vi "Perform Action.vi"(8 "error in":errorcluster, 10 "Input":variant, 11 "Virt Instrument Base in":refnum<class "Virt Instr Target Gain.lvclass">) -> (0 "error out":errorcluster, 2 "Output":variant, 3 "Virt Instrument Base out":refnum<class "Virt Instr Target Gain.lvclass">)   [LabVIEW 2023, in "HAL GOOP4.lvlib" / "Virt Instr Target Gain.lvclass"]
uses:
  Virt Instr Target Gain.lvclass
  Virt Instr Target Gain.lvclass/Virt Instr Target Gain.ctl
  Virt Instr Base/Virt Instr Base.lvclass
  af659c39-85a5-447e-8f09-7029c30334c7.vi
  <userlib>/_OpenG.lib/lvdata/lvdata.llb/openg_variant.lvlib
  Virt Instr Target/Virt Instr Target.lvclass
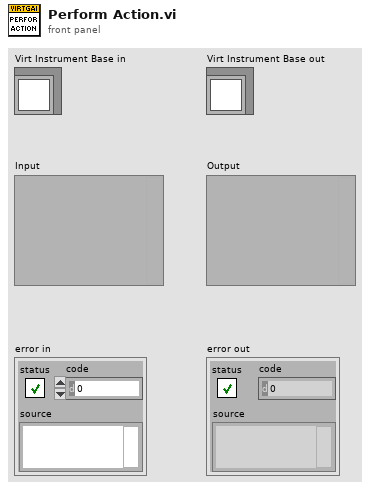
[diagram p1: front panel]
types:
  T1 = typedef "openg_variant.lvlib/Type Descriptor Enumeration__ogtk.ctl" = enum8{"<Null>", "I8", "I16", "I32", "I64", "U8", "U16", "U32", "U64", "SGL", "DBL", "EXT", "CSG", "CDB", "CXT", "0x0F", "0x10", "0x11", "0x12", "0x13", "0x14", "Enum U8", "Enum U16", "Enum U32", "Enum U64", "SGL PQ", "DBL PQ", "EXT PQ", "CSG PQ", "CDB PQ", "CXT PQ", "0x1F", "0x20", "Boolean", "0x22", "0x23", "0x24", "0x25", "0x26", "0x27", "0x28", "0x29", "0x2A", "0x2B", "0x2C", "0x2D", "0x2E", "0x2F", "String", "0x31", "Path", "Pict", "0x34", "0x35", "0x36", "DAQ", "0x38", "0x39", "0x3A", "0x3B", "0x3C", "0x3D", "0x3E", "0x3F", "Array", "0x41", "0x42", "0x43", "0x44", "0x45", "0x46", "0x47", "0x48", "0x49", "0x4A", "0x4B", "0x4C", "0x4D", "0x4E", "0x4F", "Cluster", "0x51", "0x52", "Variant", "Waveform", "0x55", "0x56", "0x57", "0x58", "0x59", "0x5A", "0x5B", "0x5C", "0x5D", "0x5E", "Fixed Point", "0x60", "0x61", "0x62", "0x63", "0x64", "0x65", "0x66", "0x67", "0x68", "0x69", "0x6A", "0x6B", "0x6C", "0x6D", "0x6E", "0x6F", "Refnum", "0x71", "0x72", "Set Collection", "Map Collection"}
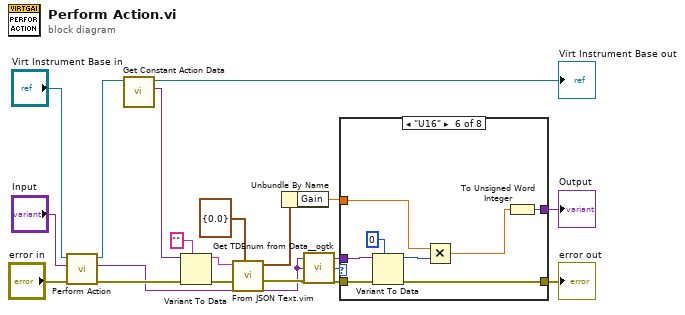
[diagram p0: block diagram]
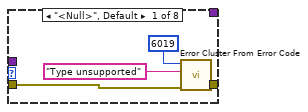
[diagram p2: hidden frame]
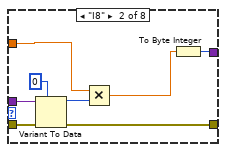
[diagram p3: hidden frame]
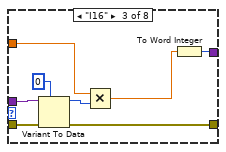
[diagram p4: hidden frame]
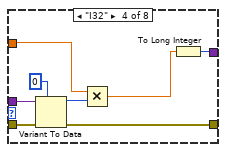
[diagram p5: hidden frame]
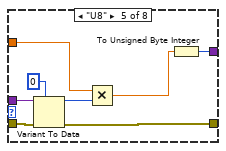
[diagram p6: hidden frame]
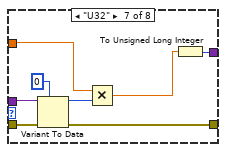
[diagram p7: hidden frame]
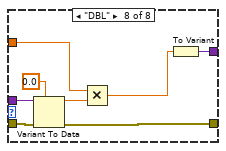
[diagram p8: hidden frame]
diagram:
  n1 = call-parent "Perform Action.vi"("error in"="error in", "Input"="Input", "Virt Instrument Base in"="Virt Instrument Base in") -> ("error out"=w5:errorcluster, "Output"=w3:variant, "Virt Instrument Base out"=w18:refnum<class "Virt Instr Target Gain.lvclass">)  [unwired: 6 in]
  n2 = call "Get Constant Action Data.vi"("Virt Instr Base in"=w18) -> ("Constant Action Data"=w12:variant, "Virt Instr Base out"=→"Virt Instrument Base out":refnum<class "Virt Instr Target Gain.lvclass">)  [unwired: 9 in]
  n3 = Variant To Data(error in=w5, type="", Variant=w12) -> (data=w11:string, error out=w10:errorcluster)
  n4 = call "From JSON Text.vim"("Data Type and Default Value"=cluster{"Gain":dbl} {"Gain"=0.0}, "error in (no error)"=w10, "JSON"=w11) -> ("error out"=w7:errorcluster, "Data out"=w8:cluster{"Gain":dbl})  [unwired: 7 in]
  n5 = Unbundle By Name(w8) -> ("Gain"=w6:dbl)
  n6 = call <userlib>:"Get TDEnum from Data__ogtk.vi"("Data"=w3) -> ("Type Descriptor Enumeration"=w4:T1)  [unwired: 4 in]
  n7 = case shown="\"U16\"" w4 {
    tunnel: w7 -> [w22 w27 w34 w45 w51 w59 w67 w76]
    tunnel: [w21 w25 w33 w42 w49 w57 w65 w75] -> w1
    tunnel: [_ w28 w36 w43 w50 w58 w66 w74] -> w2
    tunnel: w6 -> [_ w26 w35 w44 w52 w60 w68 w73]
    tunnel: w3 -> [_ w23 w31 w39 w47 w55 w63 w72]
    frame "<Null>", Default {
      n8 = call <vilib>:"Error Cluster From Error Code.vi"("error in (no error)"=w22, "error message (\"\")"="Type unsupported" ("error message (\"\")"), "error code (0)"=6019) -> ("error out"=w21:errorcluster)  [unwired: 6 in]
    }
    frame "I8" {
      n9 = Variant To Data(error in=w27, type=i8 0, Variant=w23) -> (data=w29:i8, error out=w25:errorcluster)
      n10 = Multiply(x=w26, y=w29) -> (x*y=w24:dbl)
      n11 = To Byte Integer(number=w24) -> (8bit integer=w28:i8)
    }
    frame "I16" {
      n12 = Variant To Data(error in=w34, type=i16 0, Variant=w31) -> (data=w37:i16, error out=w33:errorcluster)
      n13 = Multiply(x=w35, y=w37) -> (x*y=w32:dbl)
      n14 = To Word Integer(number=w32) -> (16bit integer=w36:i16)
    }
    frame "I32" {
      n15 = Variant To Data(error in=w45, type=0, Variant=w39) -> (data=w41:i32, error out=w42:errorcluster)
      n16 = Multiply(x=w44, y=w41) -> (x*y=w40:dbl)
      n17 = To Long Integer(number=w40) -> (32bit integer=w43:i32)
    }
    frame "U8" {
      n18 = Variant To Data(error in=w51, type=u8 0, Variant=w47) -> (data=w53:u8, error out=w49:errorcluster)
      n19 = Multiply(x=w52, y=w53) -> (x*y=w48:dbl)
      n20 = To Unsigned Byte Integer(number=w48) -> (unsigned 8bit integer=w50:u8)
    }
    frame "U16" {
      n21 = Variant To Data(error in=w59, type=u16 0, Variant=w55) -> (data=w61:u16, error out=w57:errorcluster)
      n22 = Multiply(x=w60, y=w61) -> (x*y=w56:dbl)
      n23 = To Unsigned Word Integer(number=w56) -> (unsigned 16bit integer=w58:u16)
    }
    frame "U32" {
      n24 = Variant To Data(error in=w67, type=u32 0, Variant=w63) -> (data=w69:u32, error out=w65:errorcluster)
      n25 = Multiply(x=w68, y=w69) -> (x*y=w64:dbl)
      n26 = To Unsigned Long Integer(number=w64) -> (unsigned 32bit integer=w66:u32)
    }
    frame "DBL" {
      n27 = Variant To Data(error in=w76, type=0.0, Variant=w72) -> (data=w77:dbl, error out=w75:errorcluster)
      n28 = Multiply(x=w73, y=w77) -> (x*y=w71:dbl)
      n29 = To Variant(anything=w71) -> (Variant=w74:variant)
    }
  }
  "error out" <- w1
  "Output" <- w2
